vi "Scan Name.vi"(10 "Parser State in":T1) -> (2 "Parser State":T1)   [LabVIEW 2020, in "CDM-Config.lvlib" / "Config-YAML.lvclass"]
uses:
  Config-YAML.lvclass
  Parser State.ctl
  Config-YAML.lvclass/Config-YAML.ctl
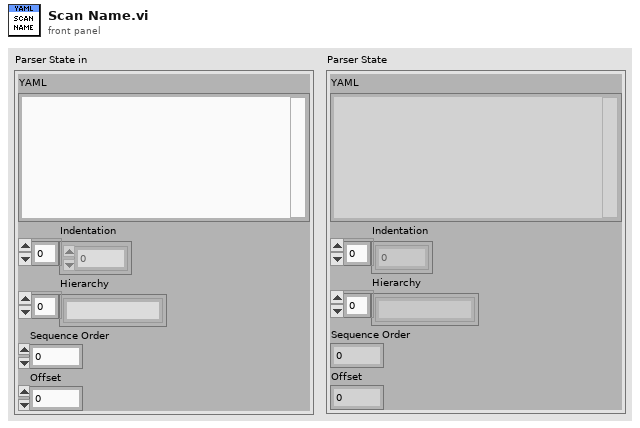
[diagram p1: front panel]
types:
  T1 = typedef "CDM-Config.lvlib/Config-YAML.lvclass/Parser State.ctl" = cluster{"YAML":string, "Indentation":i32[], "Hierarchy":string[], "Sequence Order":i32, "Offset":i32}
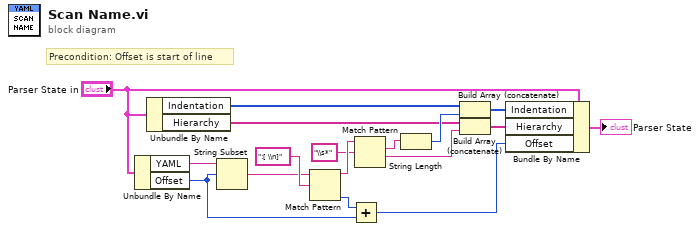
[diagram p0: block diagram]
diagram:
  # "Precondition: Offset is start of line"
  n1 = Unbundle By Name("Parser State in") -> ("YAML"=w3:string, "Offset"=w2:i32)
  n2 = Unbundle By Name("Parser State in") -> ("Indentation"=w13:i32[], "Hierarchy"=w11:string[])
  n3 = String Subset(string=w3, offset (0)=w2) -> (substring=w1:string)  [unwired: 1 in]
  n4 = Match Pattern(string=w1, regular expression=":[ \\n]") -> (before substring=w16:string, offset past match=w7:i32)  [unwired: 1 in, 2 out]
  n5 = Add(x=w7, y=w2) -> (x+y=w6:i32)
  n6 = Match Pattern(string=w16, regular expression="\\s*") -> (match substring=w14:string, after substring=w4:string)  [unwired: 1 in, 2 out]
  n7 = String Length(string=w14) -> (length=w12:i32)
  n8 = Build Array (concatenate)(w13, w12) -> (w9:i32[])
  n9 = Build Array (concatenate)(w11, w4) -> (w8:string[])
  n10 = Bundle By Name(cluster="Parser State in", "Indentation"=w9, "Hierarchy"=w8, "Offset"=w6) -> (→"Parser State":T1)
